vi "PH_SSAC.Smooth.vi"(1 "dt [fs]":dbl, 2 "Time [fs]":dbl[](array[numeric]), 3 "Frame Linear Averages [pixel]":dbl[](array[numeric])) -> (0 "Signal*Smooth":dbl[](array[numeric]) format="%0.2f")   [LabVIEW 2014, in "PH_SSAC.lvlib"]
uses:
  PH_SSAC.lvlib
  <vilib>/Analysis/2dsp.llb/Real FFT.vi
  <vilib>/Analysis/2dsp.llb/Inverse Real FFT.vi
  <vilib>/Analysis/NI_AALPro.lvlib
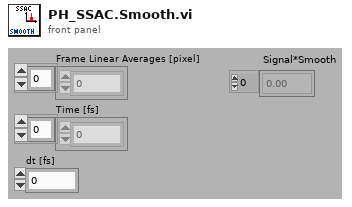
[diagram p1: front panel]
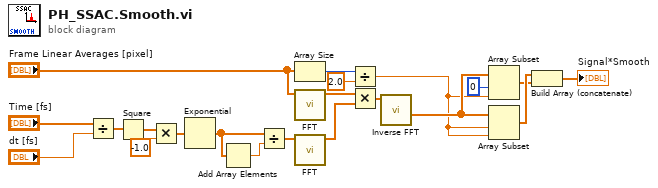
[diagram p0: block diagram]
diagram:
  n1 = Divide(x="Time [fs]", y="dt [fs]") -> (x/y=w1:dbl[])
  n2 = Square(x=w1) -> (x^2=w21:dbl[])
  n3 = Multiply(x=w21, y=-1.0) -> (x*y=w20:dbl[])
  n4 = Exponential(1:w20) -> (0:w19:dbl[])
  n5 = Add Array Elements(numeric array=w19) -> (sum=w18:dbl)
  n6 = Divide(x=w19, y=w18) -> (x/y=w16:dbl[])
  n7 = Array Size(array="Frame Linear Averages [pixel]") -> (size(s)=w12:i32)
  n8 = call-poly <vilib>:"FFT.vi"("X"="Frame Linear Averages [pixel]") -> ("FFT {X}"=w14:cdb[])  [unwired: 9 in, 1 out]
  n9 = call-poly <vilib>:"FFT.vi"("X"=w16) -> ("FFT {X}"=w15:cdb[])  [unwired: 9 in, 1 out]
  n10 = Divide(x=w12, y=2.0) -> (x/y=w8:dbl)
  n11 = Multiply(x=w14, y=w15) -> (x*y=w13:cdb[])
  n12 = call-poly <vilib>:"Inverse FFT.vi"("FFT {X}"=w13) -> ("X"=w9:dbl[])  [unwired: 9 in, 1 out]
  n13 = Array Subset(array=w9, index=0, length=w8) -> (w6:dbl[])
  n14 = Array Subset(array=w9, index=w8, length=w8) -> (w7:dbl[])
  n15 = Build Array (concatenate)(w7, w6) -> (→"Signal*Smooth":dbl[])
